vi "FM(sub).vi"(0 "File":path, 1 "Time (s)":i32=10, 5 "Baseband Frequency (Hz)":dbl=22413.793103448275, 7 "FM Deviation (Hz)":dbl=154517.79084245834, 9 "Carrier Frequency (Hz)":dbl=205410.22592152198 min=86453.20197044335, 11 "fs":dbl=10000000.0, 12 "Sample":i32=10000) -> (6 "Data":dbl[](array[numeric]), 10 "FM Signal":waveform(dbl)(graph))   [LabVIEW 2020]
uses:
  <vilib>/measure/NI_MABase.lvlib
panel:
  in  "Baseband Signal":T1(ring)
  out "Carrier Graph":waveform(dbl)(graph)
  out "Baseband Graph":waveform(dbl)(graph)
  out "Waveform Graph":waveform(dbl)(graph)
  out "Array Size":i32
  out "Data 2":dbl[](array[numeric])
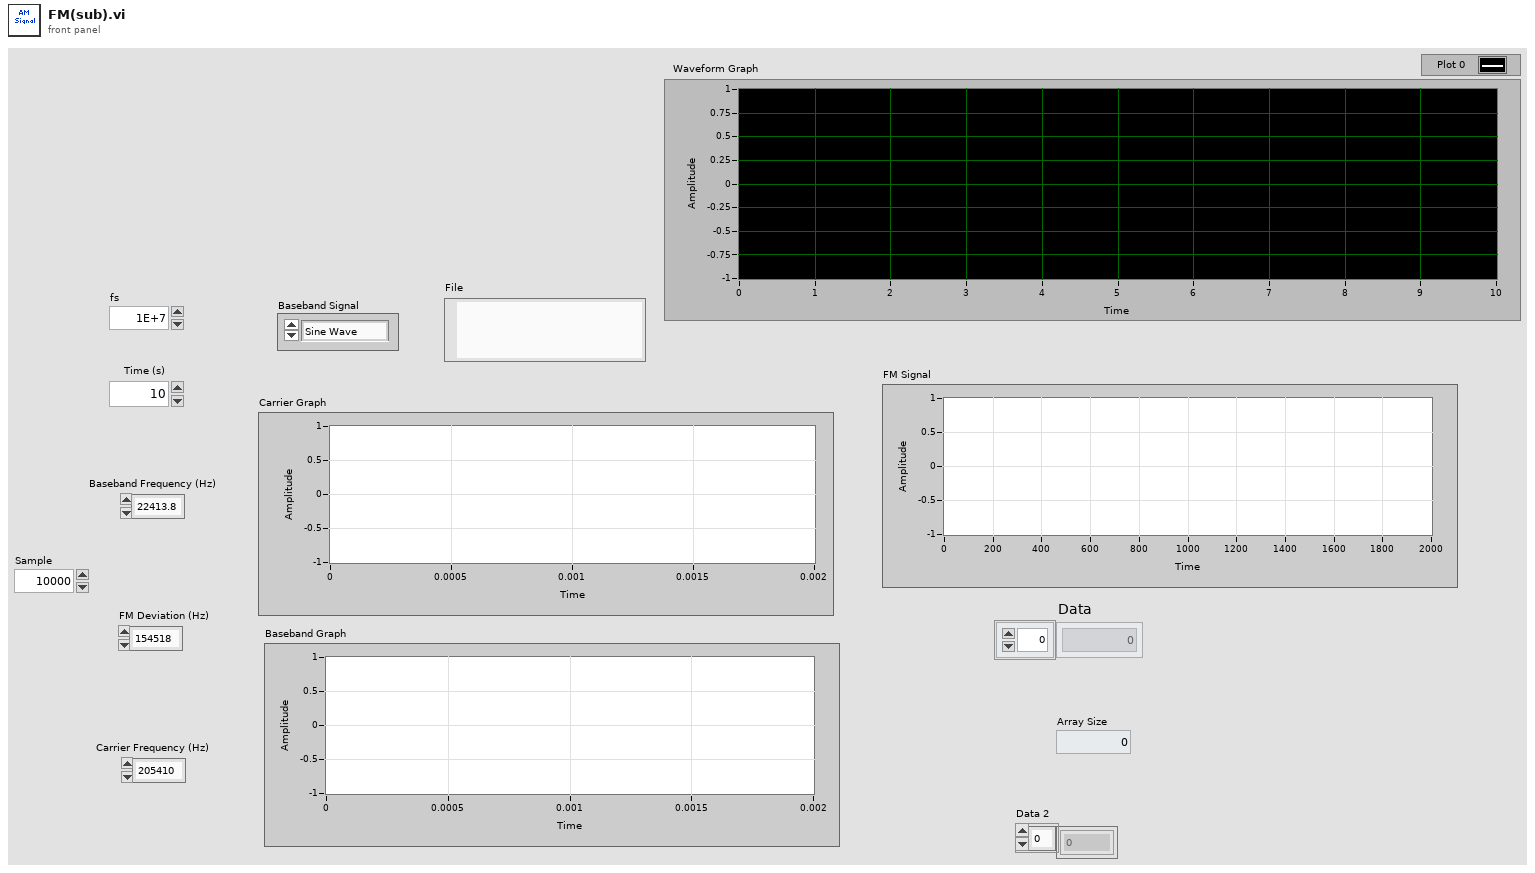
[diagram p1: front panel]
types:
  T1 = enum16{"Sine Wave", "Triangle Wave", "Square Wave", "Sawtooth Wave"}
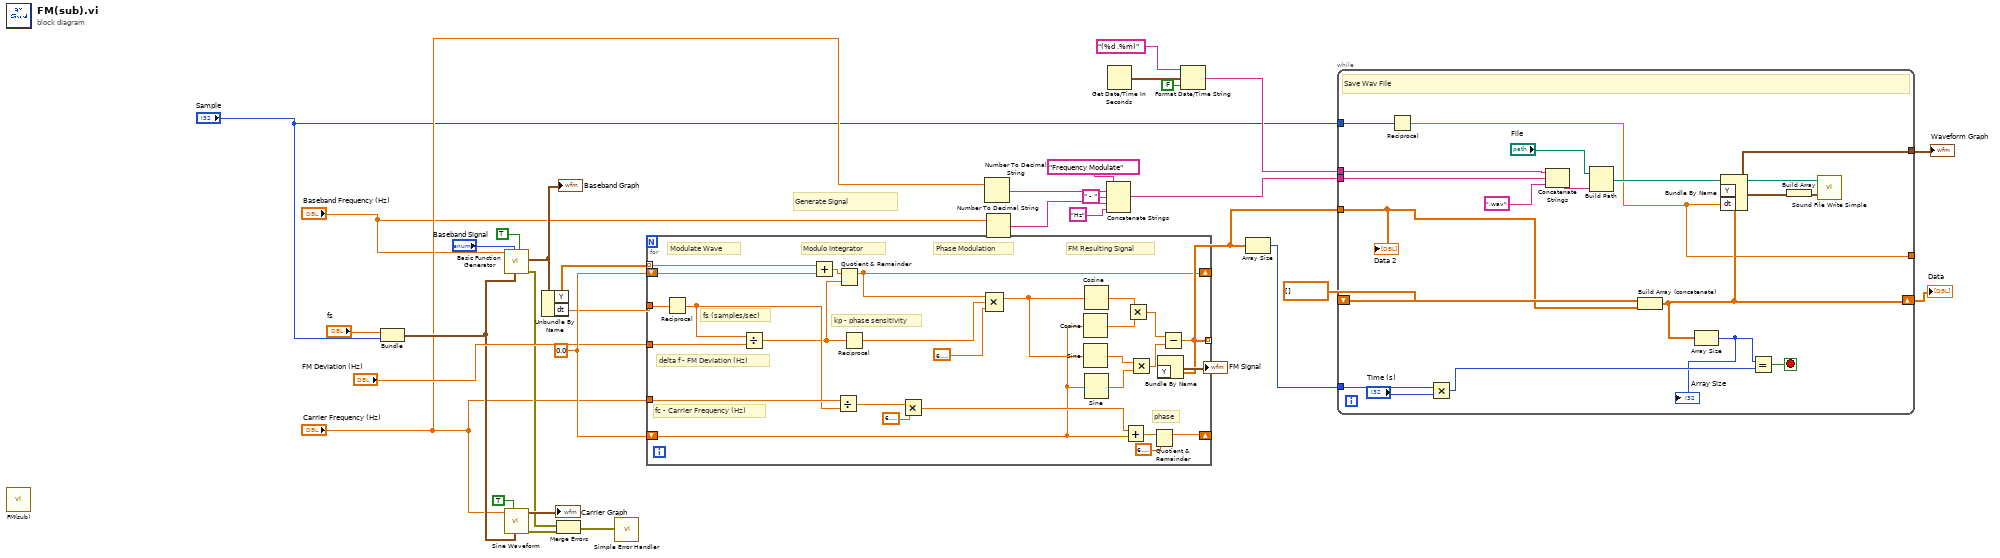
[diagram p0: block diagram]
diagram:
  w18 = 0.0
  # "Generate Signal"
  n1 = call "FM(sub).vi"() -> ()  [unwired: 14 in, 2 out]
  n2 = Bundle("fs"="fs", "Sample"="Sample") -> (w11:cluster{"fs":dbl, "Sample":i32})  [unwired: 1 in]
  n3 = call <vilib>:"Basic Function Generator.vi"("reset signal"=TRUE, "sampling info"=w11, "signal type"="Baseband Signal", "frequency"="Baseband Frequency (Hz)") -> ("error out"=w9:errorcluster, "signal out"=w6:waveform(dbl))  [unwired: 5 in, 1 out]
  "Baseband Graph" <- w6
  n4 = call <vilib>:"Sine Waveform.vi"("sampling info"=w11, "reset signal"=TRUE, "frequency"="Carrier Frequency (Hz)") -> ("error out"=w10:errorcluster, "signal out"=→"Carrier Graph":waveform(dbl))  [unwired: 7 in]
  n5 = Unbundle By Name(w6) -> ("Y"=w14:dbl[], "dt"=w16:dbl)
  n6 = Merge Errors(w9, w10) -> (w8:errorcluster)
  n7 = call <vilib>:"Simple Error Handler.vi"("error in (no error)"=w8) -> ()  [unwired: 4 in, 5 out]
  n8 = for {
    tunnel: w16 -> [w59]
    tunnel: "FM Deviation (Hz)" -> [w58]
    shift-right: [w45] -> _
    shift-left: w18 -> [w44]
    tunnel: w14 -> [w43] mode=indexing
    tunnel: "Carrier Frequency (Hz)" -> [w57]
    tunnel: [w52] -> w5 mode=indexing
    shift-right: [w48] -> _
    shift-left: w18 -> [w41]
    # "Modulate Wave"
    # "fc - Carrier Frequency (Hz)"
    # "delta f - FM Deviation (Hz)"
    # "phase"
    # "FM Resulting Signal"
    # "Phase Modulation"
    # "kp - phase sensitivity"
    # "Modulo Integrator"
    # "fs (samples/sec)"
    n9 = Reciprocal(x=w59) -> (1/x=w56:dbl)
    n10 = Divide(x=w56, y=w58) -> (x/y=w46:dbl)
    n11 = Add(x=w43, y=w44) -> (x+y=w47:dbl)
    n12 = Divide(x=w57, y=w56) -> (x/y=w54:dbl)
    n13 = Quotient & Remainder(x=w47, y=w46) -> (x-y*floor(x/y)=w45:dbl)  [unwired: 1 out]
    n14 = Reciprocal(x=w46) -> (1/x=w35:dbl)
    n15 = Multiply(x=w54, y=6.283185307179586) -> (x*y=w51:dbl)
    n16 = Compound Arithmetic op=MULTIPLY(w45, w35, 6.283185307179586) -> (w36:dbl)
    n17 = Cosine(x=w41) -> (cos(x)=w38:dbl)
    n18 = Sine(x=w36) -> (sin(x)=w37:dbl)
    n19 = Cosine(x=w36) -> (cos(x)=w39:dbl)
    n20 = Sine(x=w41) -> (sin(x)=w40:dbl)
    n21 = Add(x=w51, y=w41) -> (x+y=w50:dbl)
    n22 = Multiply(x=w39, y=w38) -> (x*y=w53:dbl)
    n23 = Multiply(x=w37, y=w40) -> (x*y=w42:dbl)
    n24 = Quotient & Remainder(x=w50, y=6.283185307179586) -> (x-y*floor(x/y)=w48:dbl)  [unwired: 1 out]
    n25 = Subtract(x=w53, y=w42) -> (x-y=w52:dbl)
  }
  n26 = Number To Decimal String(number="Carrier Frequency (Hz)") -> (decimal integer string=w32:string)  [unwired: 1 in]
  n27 = Number To Decimal String(number="Baseband Frequency (Hz)") -> (decimal integer string=w21:string)  [unwired: 1 in]
  n28 = Concatenate Strings("Frequency Modulate", w32, " - " ("string"), w21, "Hz" ("string")) -> (w27:string)
  n29 = Get Date/Time In Seconds() -> (seconds since 1Jan1904=w28:timestamp)
  n30 = Bundle By Name("Y"=w5) -> (→"FM Signal":waveform(dbl))  [unwired: 1 in]
  n31 = Format Date/Time String(time format string (%c)="(%d .%m)", seconds (now)=w28, UTC format=FALSE) -> (date/time string=w31:string)
  n32 = Array Size(array=w5) -> (size(s)=w23:i32)
  n33 = while {
    tunnel: "Sample" -> [w77]
    tunnel: w5 -> [w74]
    shift-right: [w73] -> w26
    shift-left: dbl[] [] ("Array") -> [w75]
    tunnel: w23 -> [w69]
    tunnel: [w66] -> _
    tunnel: [w64] -> w25
    tunnel: w27 -> [w63]
    tunnel: w31 -> [w61]
    stop <- w72 stop-if-true
    # "Save Wav File"
    n34 = Reciprocal(x=w77) -> (1/x=w66:dbl)
    n35 = Multiply(x=w69, y="Time (s)") -> (x*y=w71:i32)
    n36 = Concatenate Strings(w61, w63, ".wav") -> (w65:string)
    n37 = Build Path(base path="File", name or relative path=w65) -> (appended path=w76:path)
    n38 = Build Array (concatenate)(w75, w74) -> (w73:dbl[])
    n39 = Array Size(array=w73) -> (size(s)=w70:i32)
    "Array Size" <- w70
    n40 = Bundle By Name("Y"=w73, "dt"=w66) -> (w64:waveform(dbl))  [unwired: 1 in]
    n41 = Equal?(x=w70, y=w71) -> (x = y?=w72:bool)
    n42 = Build Array(w64) -> (w67:waveform(dbl)[])
    n43 = call <vilib>:"Sound File Write Simple.vi"("data"=w67, "path"=w76) -> ()  [unwired: 8 in, 2 out]
    "Data 2" <- w74
  }
  "Data" <- w26
  "Waveform Graph" <- w25
